vi "Stop Test.vi"(8 "error in (no error)":errorcluster, 11 "Report Plugin In":refnum<class "Report Plugin.lvclass">) -> (0 "error out":errorcluster, 3 "Report Plugin Out":refnum<class "Report Plugin.lvclass">)   [LabVIEW 2020, in "Report Plugin.lvclass"]
uses:
  Report Plugin.lvclass
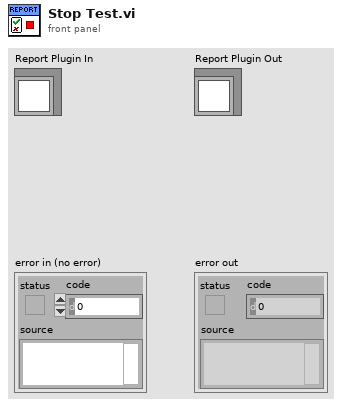
[diagram p1: front panel]
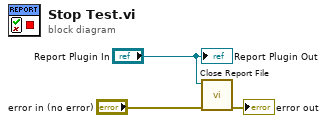
[diagram p0: block diagram]
diagram:
  n1 = call-dynamic "Close Report File.vi"("error in (no error)"="error in (no error)", "Report In"="Report Plugin In") -> ("error out"=→"error out":errorcluster)  [unwired: 8 in, 1 out]
  "Report Plugin Out" <- "Report Plugin In"
